vi "Configure HDI.vi"(8 "error in (no error)":errorcluster, 11 "WorkTable Class in":refnum<class "WorkTable Class.lvclass">) -> (0 "error out":errorcluster, 3 "WorkTable Class out":refnum<class "WorkTable Class.lvclass">)   [LabVIEW 2011, in "WorkTable Class.lvclass"]
uses:
  WorkTable Class.lvclass
  <vilib>/Utility/config.llb/Read Key (Double).vi
  <vilib>/Utility/config.llb/NI_LVConfig.lvlib
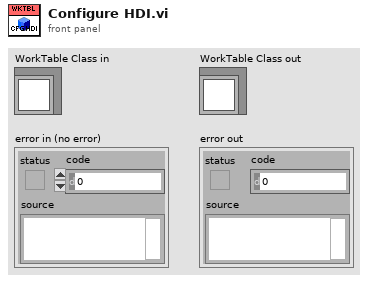
[diagram p1: front panel]
types:
  T1 = typedef "NI_LVConfig.lvlib/Config Data RefNum.ctl" = refnum<k1>
  T2 = cluster{"HDI Assembly State":enum16{"Empty", "Populated"}, "HDI Type":enum16{"HDI", "Polyimide"}, "Vacuum":bool, "Fidicual Locations":cluster{"x":dbl, "y":dbl, "z":dbl}[]}[]
  T3 = cluster{"HDI Assembly State":enum16{"Empty", "Populated"}, "HDI Type":enum16{"HDI", "Polyimide"}, "Vacuum":bool, "Fidicual Locations":cluster{"x":dbl, "y":dbl, "z":dbl}[]}
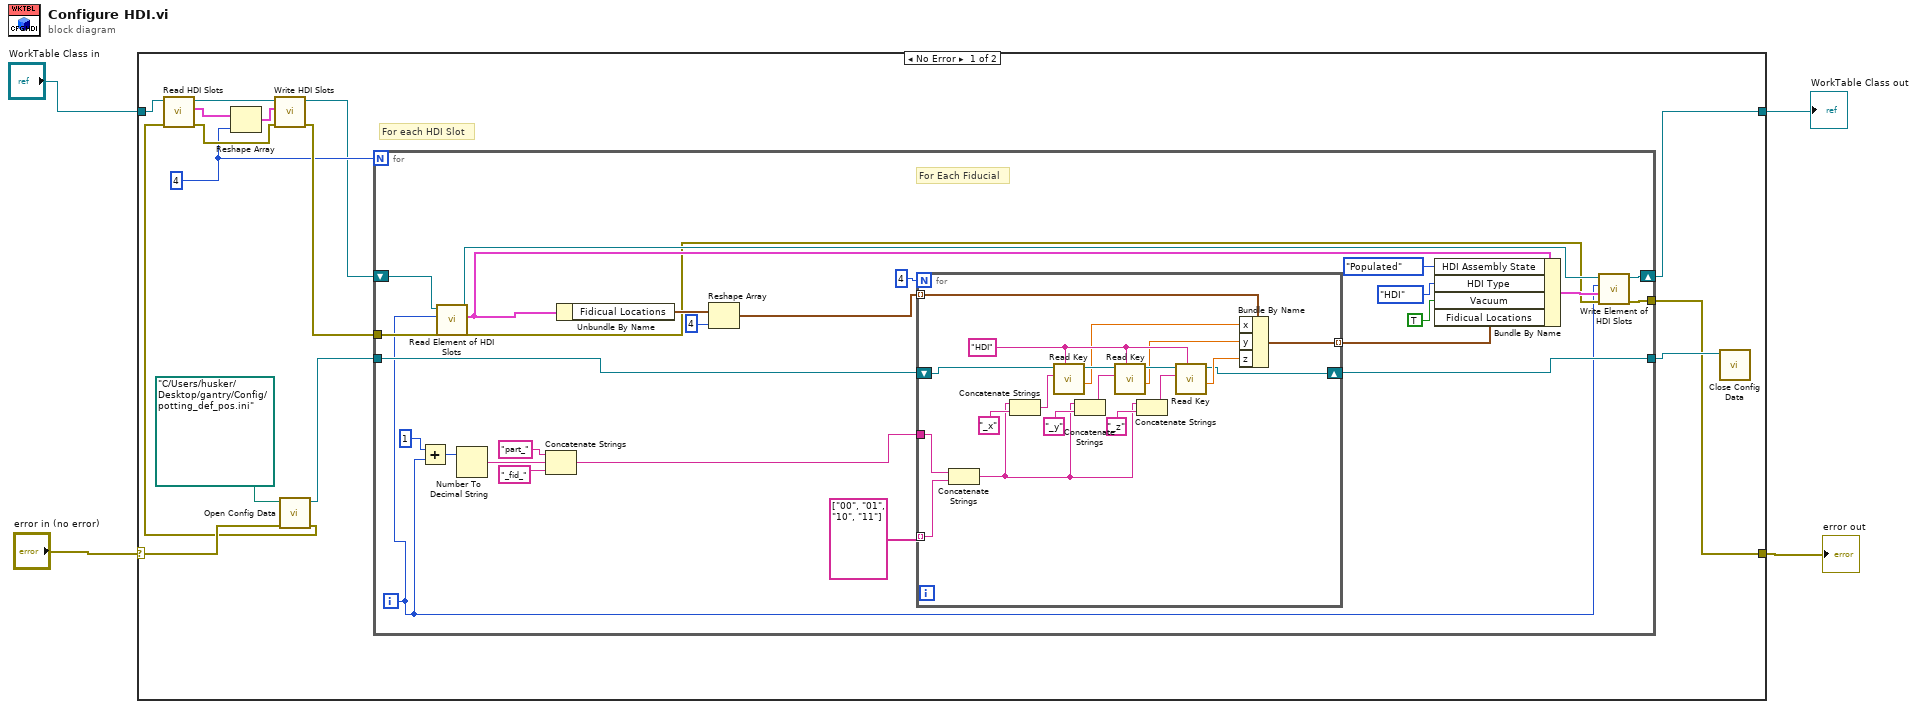
[diagram p0: block diagram]
diagram:
  n1 = case shown="No Error" "error in (no error)" {
    selector: "error in (no error)" -> [w18 w66]
    tunnel: [w7 w66] -> w2
    tunnel: [w11 w65] -> w3
    tunnel: "WorkTable Class in" -> [w15 w65]
    frame No Error {
      w6 = 4 ("dimension size")
      # "For each HDI Slot"
      n2 = call <vilib>:"Open Config Data.vi"("error in (no error)"=w18, "configuration file path"=path "C:/Users/husker/Desktop/gantry/Config/potting_def_pos.ini") -> ("error out"=w10:errorcluster, "refnum"=w17:T1)  [unwired: 7 in, 1 out]
      n3 = call-dynamic "Read HDI Slots.vi"("error in (no error)"=w10, "WorkTable Class in"=w15) -> ("error out"=w9:errorcluster, "HDI Slots"=w14:T2, "WorkTable Class out"=w12:refnum<class "WorkTable Class.lvclass">)  [unwired: 7 in]
      n4 = Reshape Array(w14, w6) -> (w13:T2)
      n5 = call-dynamic "Write HDI Slots.vi"("error in (no error)"=w9, "HDI Slots"=w13, "WorkTable Class in"=w12) -> ("error out"=w8:errorcluster, "WorkTable Class out"=w5:refnum<class "WorkTable Class.lvclass">)  [unwired: 7 in]
      n6 = for {
        N: w6 -> [_]
        tunnel: w17 -> [w39]
        tunnel: [w38] -> w16
        tunnel: w8 -> [w25]
        tunnel: [w23] -> w7
        shift-right: [w26] -> w11
        shift-left: w5 -> [w20]
        i -> [w21]
        # "For Each Fiducial"
        n7 = Add(x=1, y=w21) -> (x+y=w44:i32)
        n8 = call-dynamic "Read Element of HDI Slots.vi"("error in (no error)"=w25, "index"=w21, "WorkTable Class in"=w20) -> ("error out"=w24:errorcluster, "HDI Slot"=w32:T3, "WorkTable Class out"=w33:refnum<class "WorkTable Class.lvclass">)  [unwired: 6 in]
        n9 = Number To Decimal String(number=w44) -> (decimal integer string=w42:string)  [unwired: 1 in]
        n10 = Concatenate Strings("part_" ("string"), w42, "_fid_" ("string")) -> (w40:string)
        n11 = Unbundle By Name(w32) -> ("Fidicual Locations"=w36:cluster{"x":dbl, "y":dbl, "z":dbl}[])
        n12 = Reshape Array(w36, 4 ("dimension size")) -> (w34:cluster{"x":dbl, "y":dbl, "z":dbl}[])
        n13 = for {
          N: 4 -> [_]
          tunnel: string[] ["00", "01", "10", "11"] -> [w63] mode=indexing
          tunnel: w40 -> [w64]
          shift-right: [w49] -> w38
          shift-left: w39 -> [w48]
          tunnel: w34 -> [w47] mode=indexing
          tunnel: [w46] -> w31 mode=indexing
          w60 = "HDI" ("section")
          n14 = Concatenate Strings(w64, w63) -> (w55:string)
          n15 = Concatenate Strings(w55, "_x" ("string")) -> (w58:string)
          n16 = call-poly <vilib>:"Read Key.vi"("section"=w60, "key"=w58, "refnum"=w48) -> ("value"=w50:dbl, "refnum out"=w62:T1)  [unwired: 5 in, 2 out]
          n17 = Concatenate Strings(w55, "_y" ("string")) -> (w54:string)
          n18 = call-poly <vilib>:"Read Key.vi"("section"=w60, "key"=w54, "refnum"=w62) -> ("value"=w51:dbl, "refnum out"=w61:T1)  [unwired: 5 in, 2 out]
          n19 = Concatenate Strings(w55, "_z" ("string")) -> (w53:string)
          n20 = call-poly <vilib>:"Read Key.vi"("section"=w60, "key"=w53, "refnum"=w61) -> ("value"=w52:dbl, "refnum out"=w49:T1)  [unwired: 5 in, 2 out]
          n21 = Bundle By Name(cluster=w47, "x"=w50, "y"=w51, "z"=w52) -> (w46:cluster{"x":dbl, "y":dbl, "z":dbl})
        }
        n22 = Bundle By Name(cluster=w32, "HDI Assembly State"=enum16{"Empty", "Populated"}."Populated", "HDI Type"=enum16{"HDI", "Polyimide"}."HDI", "Vacuum"=TRUE, "Fidicual Locations"=w31) -> (w30:T3)
        n23 = call-dynamic "Write Element of HDI Slots.vi"("error in (no error)"=w24, "HDI Slot"=w30, "index"=w21, "WorkTable Class in"=w33) -> ("error out"=w23:errorcluster, "WorkTable Class out"=w26:refnum<class "WorkTable Class.lvclass">)  [unwired: 6 in]
      }
      n24 = call <vilib>:"Close Config Data.vi"("refnum"=w16) -> ()  [unwired: 9 in, 2 out]
    }
    frame Error {
    }
  }
  "WorkTable Class out" <- w3
  "error out" <- w2
